vi "Engine-RPC-PWMPumpA.vi"(8 "Error In":errorcluster, 11 "DSI Reference":refnum<class "DCM-DSI.lvclass">) -> (0 "Error Out":errorcluster, 3 "DSI Reference":refnum<class "DCM-DSI.lvclass">)   [LabVIEW 2016, in "DSI-RT.lvlib"]
uses:
  DSI-RT.lvlib
  Classes/DCM-DSI/DCM-DSI.lvclass
  <vilib>/Powertrain Controls/Device Drivers/DCM/HH/FPGA/Mode.ctl
  <vilib>/Powertrain Controls/Device Drivers/DCM/HH/RT/Setup.ctl
  <vilib>/Powertrain Controls/Device Drivers/DCM/Rev0/FPGA/Digital Channel.ctl
  <vilib>/Powertrain Controls/Device Drivers/DCM/HH/RT/Angle Control.ctl
  Shared/Typedefs/Engine-RPC-PWM-Indicators.ctl
  <vilib>/addons/Software Calibration Management/xSCM/Controls/TBL1D.ctl
  <vilib>/Powertrain Controls/Device Drivers/DCM/Rev0/RT/DCM - RT.lvclass/DCM - RT.ctl
  <vilib>/Powertrain Controls/Device Drivers/DCM/HH/RT/Mode.ctl
  <vilib>/Powertrain Controls/Device Drivers/DCM/Rev0/RT/Read HH Mode.vi
  Classes/DCM-DSI/Read Channels.vi
  Classes/DCM-DSI/Read System ADC.vi
  Classes/DCM-DSI/Read dt.vi
  Classes/DCM-DSI/Write HH Command.vi
  Classes/DCM-DSI/Write HH Chans Used.vi
  Classes/DCM-DSI/Read DCM Ref.vi
  <vilib>/addons/Software Calibration Management/xSCM/CalPoint.xnode
  <vilib>/addons/Software Calibration Management/xSCM/FaultPoint.xnode
  <vilib>/Powertrain Controls/Device Drivers/DCM/Rev0/RT/DCM - RT.lvclass
  <vilib>/Powertrain Controls/Device Drivers/DCM/HH/FPGA/DCM - FPGA - HH.lvlib
  <vilib>/addons/Software Calibration Management/xSCM/ni_scm.dll
  <vilib>/addons/Software Calibration Management/xSCM/SCM-API.lvlib
  <vilib>/Powertrain Controls/Device Drivers/DCM/HH/RT/DCM - RT - HH.lvlib
  <vilib>/Powertrain Controls/Device Drivers/DCM/Rev0/FPGA/DCM - FPGA.lvlib
  Shared/DSI-Shared.lvlib
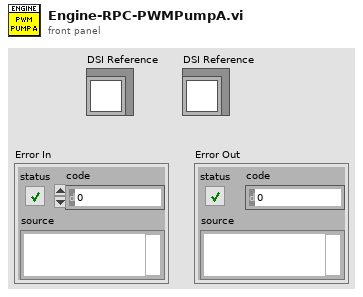
[diagram p1: front panel]
types:
  T1 = typedef "DSI-Shared.lvlib/Engine-RPC-PWM-Indicators.ctl" = cluster{"IMV":cluster{"Current_Calc":sgl, "DutyCyc_PIDOut":sgl, "DutyCyc_MaxCalc":sgl, "DutyCyc_Des":sgl}, "HPV":cluster{"Current_Calc":sgl, "DutyCyc_TblOut":sgl, "DutyCyc_MaxCalc":sgl, "DutyCyc_Des":sgl}}
  T2 = typedef "DCM - RT - HH.lvlib/Setup.ctl" = cluster{"Mode":T3, "Digital Input":T4, "Polarity":bool, "Frequency [Hz]":sgl, "Duty Cycle [%]":sgl, "TDC Offset [CAD]":sgl, "Window Start [DBTDC]":sgl, "Window End [DBTDC]":sgl, "Angles":T5[], "Skip Fire":bool, "Skip Fire Index":u8}
  T3 = typedef "DCM - FPGA - HH.lvlib/Mode.ctl" = enum8{"Off", "Direct", "Pulse Width Modulation", "Engine Position Tracking"}
  T4 = typedef "DCM - FPGA.lvlib/Digital Channel.ctl" = enum8{"Unused", "User OS", "Diff IO 1", "Diff IO 2", "Diff IO 3", "Diff IO 4", "Diff IO 5", "Diff IO 6", "Diff IO 7", "Diff IO 8", "Aux 1", "Aux 2", "Aux 3", "Aux 4", "Aux 5", "Aux 6", "Aux 7", "Aux 8", "Aux 9", "Aux 10", "Aux 11", "Aux 12", "Aux 13", "Aux 14", "Aux 15", "Aux 16"}
  T5 = typedef "DCM - RT - HH.lvlib/Angle Control.ctl" = cluster{"Enable":bool, "Location [DBTDC]":sgl, "Duration [s]":sgl}
  T6 = cluster{"PID_Kp":sgl, "PID_Ti":sgl, "PID_Td":sgl, "PID_FF":sgl, "Non-PID_FF":sgl, "PID_Min":sgl, "PID_Max":sgl}
  T7 = typedef "DCM-DSI.lvclass/Channel.ctl" = cluster{"Name":string, "Unit":string, "Value":sgl}
  T8 = typedef "DCM - RT.lvclass/System ADC.ctl" = cluster{"AI 1 [V]":sgl, "AI 2 [V]":sgl, "AI 3 [V]":sgl, "AI 4 [V]":sgl, "AI 5 [V]":sgl, "AI 6 [V]":sgl, "AI 7 [V]":sgl, "AI 8 [V]":sgl, "AI 9 [V]":sgl, "AI 10 [V]":sgl, "AI 11 [V]":sgl, "AI 12 [V]":sgl, "Temp HH 1-6 [C]":sgl, "Temp HH 7-12 [C]":sgl, "Temp DI A [C]":sgl, "Temp DI Zener A [C]":sgl, "Temp DI B [C]":sgl, "Temp DI Zener B [C]":sgl, "Temp CPU [C]":sgl, "Temp Fan Intake [C]":sgl, "Temp Secondary A [C]":sgl, "Temp Primary A [C]":sgl, "Temp Boost B [C]":sgl, "Primary Range [V]":sgl, "Primary A1A2 [V]":sgl, "Primary A3A4 [V]":sgl, "Primary B3B4 [V]":sgl, "Primary B1B2 [V]":sgl, "Secondary A1A2 [V]":sgl, "Secondary A3A4 [V]":sgl, "Secondary B3B4 [V]":sgl, "Secondary B1B2 [V]":sgl, "Ext HV A [V]":sgl, "Ext HV B [V]":sgl, "FET Driver [V]":sgl, "Fan [V]":sgl, "Battery [V]":sgl, "DRVP [V]":sgl, "Key [V]":sgl, "DI Zener A [V]":sgl, "DI Zener B [V]":sgl, "Pump Zener A [V]":sgl, "Pump Zener B [V]":sgl, "MPRD [V]":sgl}
  T9 = cluster{"IMV":cluster{"PWMFreq":sgl, "NomResistance":sgl, "DutyCyc_Max":sgl, "Min Duty Cycle":sgl, "DutyCycle_ManE":bool, "DutyCycle_Man":sgl}, "HPV":cluster{"PWMFreq":sgl, "NomResistance":sgl, "DutyCyc_Max":sgl, "Min Duty Cycle":sgl, "DutyCycle_ManE":bool, "DutyCycle_Man":sgl}}
  T10 = typedef "SCM-API.lvlib/TBL1D.ctl" = cluster{"X":sgl[], "Y":sgl[]}
  T11 = cluster{"PWMFreq":sgl, "NomResistance":sgl, "DutyCyc_Max":sgl, "Min Duty Cycle":sgl, "DutyCycle_ManE":bool, "DutyCycle_Man":sgl}
  T12 = cluster{"Current_Calc":sgl, "DutyCyc_TblOut":sgl, "DutyCyc_MaxCalc":sgl, "DutyCyc_Des":sgl}
  T13 = cluster{"Enable LS Channel":bool, "Freq [Hz]":sgl, "DutyCyc [%]":sgl}
  T14 = cluster{"Current_Calc":sgl, "DutyCyc_PIDOut":sgl, "DutyCyc_MaxCalc":sgl, "DutyCyc_Des":sgl}
  T15 = cluster{"ProportionalAction":sgl, "IntegralAction":sgl, "DerivativeAction":sgl}
  T16 = typedef "DCM - RT - HH.lvlib/Mode.ctl" = enum16{"Off", "Lowside", "Highside", "PFI", "Full H", "3-Phase"}
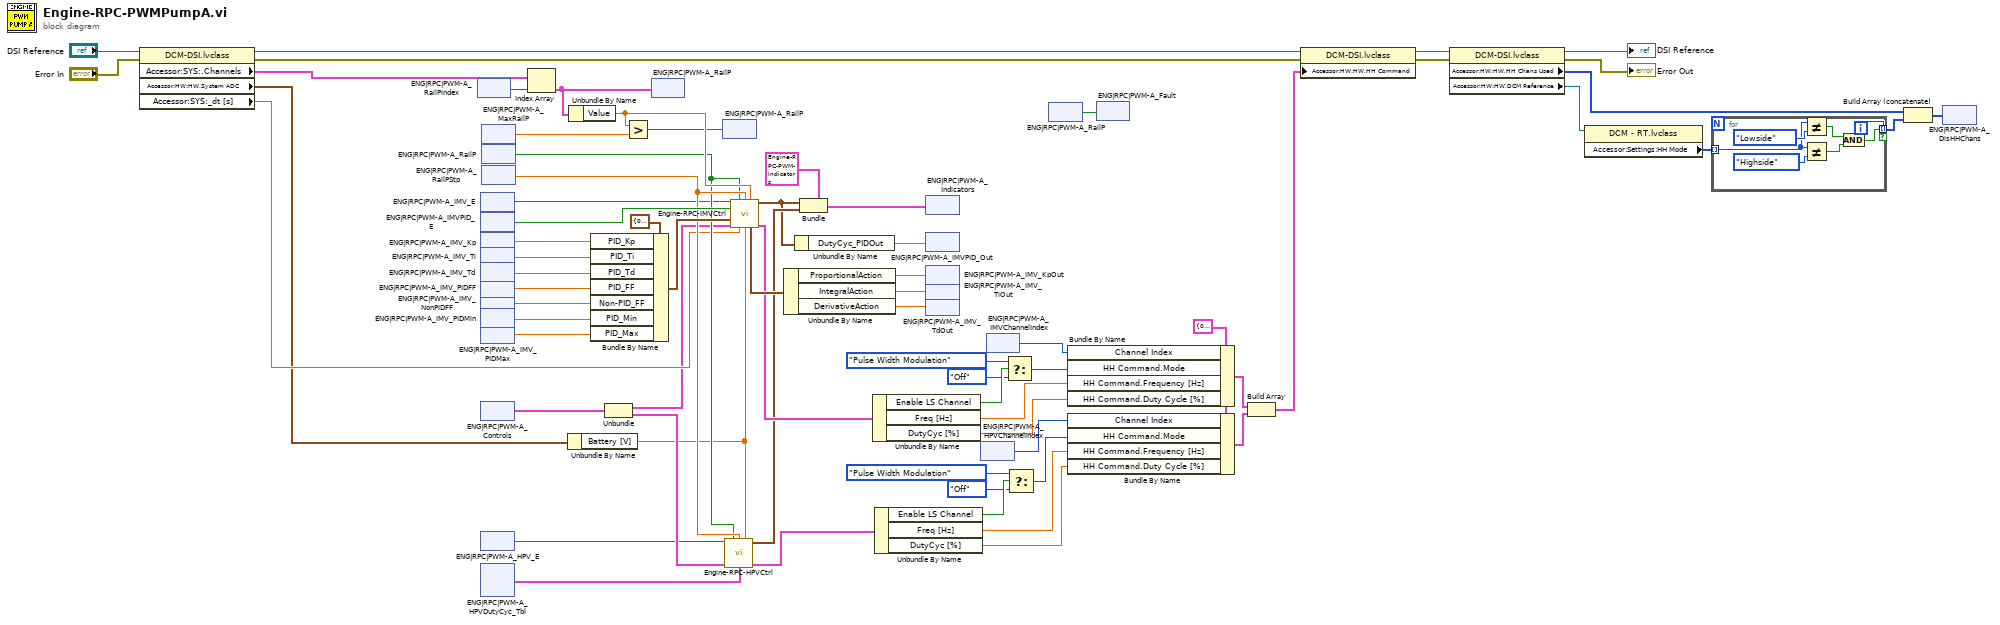
[diagram p0: block diagram]
diagram:
  w12 = cluster{"Channel Index":i32, "HH Command":T2} {"Channel Index"=0, "HH Command"={"Mode"=enum."Off", "Digital Input"=enum."Unused", "Polarity"=FALSE, "Frequency [Hz]"=0.0, "Duty Cycle [%]"=0.0, "TDC Offset [CAD]"=0.0, "Window Start [DBTDC]"=0.0, "Window End [DBTDC]"=0.0, "Angles"=[], "Skip Fire"=FALSE, "Skip Fire Index"=0}} ("HH Command")
  n1 = property class="DCM-DSI.lvclass"(reference="DSI Reference", error in="Error In") -> (reference out=w9:refnum<class "DCM-DSI.lvclass">, error out=w8:errorcluster, "Accessor:SYS:.Channels"=w13:T7[], "Accessor:HW:HW.System ADC"=w29:T8, "Accessor:SYS:_dt [s]"=w30:sgl)
  n2 = xnode "ENG|RPC|PWM-A_RailPIndex"() -> ("Value"=w39:i32)
  n3 = xnode "ENG|RPC|PWM-A_IMV_E"() -> ("Value"=w23:bool)
  n4 = xnode "ENG|RPC|PWM-A_IMVPID_E"() -> ("Value"=w36:bool)
  n5 = xnode "ENG|RPC|PWM-A_IMV_Kp"() -> ("Value"=w52:sgl)
  n6 = xnode "ENG|RPC|PWM-A_IMV_Ti"() -> ("Value"=w53:sgl)
  n7 = xnode "ENG|RPC|PWM-A_IMV_Td"() -> ("Value"=w54:sgl)
  n8 = xnode "ENG|RPC|PWM-A_IMV_PIDFF"() -> ("Value"=w55:sgl)
  n9 = xnode "ENG|RPC|PWM-A_IMV_NonPIDFF"() -> ("Value"=w56:sgl)
  n10 = xnode "ENG|RPC|PWM-A_IMV_PIDMin"() -> ("Value"=w57:sgl)
  n11 = xnode "ENG|RPC|PWM-A_IMV_PIDMax"() -> ("Value"=w58:sgl)
  n12 = xnode "ENG|RPC|PWM-A_Controls"() -> ("Value"=w22:T9)
  n13 = xnode "ENG|RPC|PWM-A_HPV_E"() -> ("Value"=w17:bool)
  n14 = xnode "ENG|RPC|PWM-A_HPVDutyCyc_Tbl"() -> ("Value"=w18:T10)
  n15 = xnode "ENG|RPC|PWM-A_MaxRailP"() -> ("Value"=w33:sgl)
  n16 = xnode "ENG|RPC|PWM-A_RailP"() -> ("Fault"=w31:bool)
  n17 = xnode "ENG|RPC|PWM-A_RailPStp"() -> ("Value"=w35:sgl)
  n18 = Index Array(array=w13, index=w39) -> (element=w38:T7)
  n19 = Unbundle By Name(w29) -> ("Battery [V]"=w19:sgl)
  n20 = Unbundle By Name(w38) -> ("Value"=w34:sgl)
  n21 = Bundle By Name(cluster=T6 {"PID_Kp"=0.0, "PID_Ti"=0.01, "PID_Td"=0.0, "PID_FF"=0.0, "Non-PID_FF"=0.0, "PID_Min"=-100.0, "PID_Max"=100.0} ("PID Settings"), "PID_Kp"=w52, "PID_Ti"=w53, "PID_Td"=w54, "PID_FF"=w55, "Non-PID_FF"=w56, "PID_Min"=w57, "PID_Max"=w58) -> (w40:T6)
  n22 = Unbundle(w22) -> ("IMV"=w21:T11, "HPV"=w20:T11)
  n23 = Greater?(x=w34, y=w33) -> (0:w32:bool)
  n24 = xnode "ENG|RPC|PWM-A_RailP"("Value"=w38) -> ()
  n25 = xnode "ENG|RPC|PWM-A_RailP"("Fault"=w32) -> ()
  n26 = call "Engine-RPC-HPVCtrl.vi"("Control Enable"=w17, "Fault Input"=w31, "RailP Setpoint"=w35, "Battery [V]"=w19, "Output Management Controls"=w20, "Open Loop DC Table"=w18) -> ("Output"=w24:T12, "LS Output"=w37:T13)  [unwired: 8 in]
  n27 = call "Engine-RPC-IMVCtrl.vi"("Control Enable"=w23, "Fault Input"=w31, "Rail Press Setpoint"=w35, "Rail Pressure"=w34, "PID Enable"=w36, "PID Settings"=w40, "Output Management Controls"=w21, "dt (s)"=w30, "Battery [V]"=w19) -> ("Output"=w14:T14, "PID_Action_Output"=w59:T15, "LS Output"=w45:T13)  [unwired: 4 in]
  n28 = Unbundle By Name(w59) -> ("ProportionalAction"=w2:sgl, "IntegralAction"=w3:sgl, "DerivativeAction"=w4:sgl)
  n29 = Unbundle By Name(w14) -> ("DutyCyc_PIDOut"=w1:sgl)
  n30 = Bundle(cluster=T1 {"IMV"={"Current_Calc"=0.0, "DutyCyc_PIDOut"=0.7671859, "DutyCyc_MaxCalc"=0.0, "DutyCyc_Des"=0.7671859}, "HPV"={"Current_Calc"=0.0, "DutyCyc_TblOut"=0.7671859, "DutyCyc_MaxCalc"=0.0, "DutyCyc_Des"=0.7671859}} ("PWM-B_Indicators"), "IMV"=w14, "HPV"=w24) -> (w5:T1)
  n31 = Unbundle By Name(w45) -> ("Enable LS Channel"=w50:bool, "Freq [Hz]"=w48:sgl, "DutyCyc [%]"=w47:sgl)
  n32 = Unbundle By Name(w37) -> ("Enable LS Channel"=w46:bool, "Freq [Hz]"=w27:sgl, "DutyCyc [%]"=w26:sgl)
  n33 = xnode "ENG|RPC|PWM-A_Indicators"("Value"=w5) -> ()
  n34 = xnode "ENG|RPC|PWM-A_IMVPID_Out"("Value"=w1) -> ()
  n35 = xnode "ENG|RPC|PWM-A_IMV_KpOut"("Value"=w2) -> ()
  n36 = xnode "ENG|RPC|PWM-A_IMV_TiOut"("Value"=w3) -> ()
  n37 = xnode "ENG|RPC|PWM-A_IMV_TdOut"("Value"=w4) -> ()
  n38 = xnode "ENG|RPC|PWM-A_HPVChannelIndex"() -> ("Value"=w15:i32)
  n39 = xnode "ENG|RPC|PWM-A_IMVChannelIndex"() -> ("Value"=w16:i32)
  n40 = Select(t=Mode."Pulse Width Modulation" ("Mode"), s=w50, f=Mode."Off" ("Mode")) -> (s? t:f=w49:T3)
  n41 = Select(t=Mode."Pulse Width Modulation" ("Mode"), s=w46, f=Mode."Off" ("Mode")) -> (s? t:f=w28:T3)
  n42 = xnode "ENG|RPC|PWM-A_RailP"() -> ("Fault"=w10:bool)
  n43 = Bundle By Name(cluster=w12, "Channel Index"=w16, "HH Command.Mode"=w49, "HH Command.Frequency [Hz]"=w48, "HH Command.Duty Cycle [%]"=w47) -> (w11:cluster{"Channel Index":i32, "HH Command":T2})
  n44 = Bundle By Name(cluster=w12, "Channel Index"=w15, "HH Command.Mode"=w28, "HH Command.Frequency [Hz]"=w27, "HH Command.Duty Cycle [%]"=w26) -> (w25:cluster{"Channel Index":i32, "HH Command":T2})
  n45 = xnode "ENG|RPC|PWM-A_Fault"("Value"=w10) -> ()
  n46 = Build Array(w11, w25) -> (w7:cluster{"Channel Index":i32, "HH Command":T2}[])
  n47 = property class="DCM-DSI.lvclass"(reference=w9, error in=w8, "Accessor:HW:HW.HH Command"=w7) -> (reference out=w66:refnum<class "DCM-DSI.lvclass">, error out=w65:errorcluster)
  n48 = property class="DCM-DSI.lvclass"(reference=w66, error in=w65) -> (reference out=→"DSI Reference":refnum<class "DCM-DSI.lvclass">, error out=→"Error Out":errorcluster, "Accessor:HW:HW.HH Chans Used"=w61:i32[], "Accessor:HW:HW.DCM Reference"=w62:refnum<class "DCM - RT.lvclass">)
  n49 = property class="DCM - RT.lvclass"(reference=w62) -> ("Accessor:Settings:HH Mode"=w64:T16[])  [unwired: 1 in, 2 out]
  n50 = for {
    tunnel: [w76] -> w60 mode=indexing if=w74
    tunnel: w64 -> [w71] mode=indexing
    i -> [w76]
    n51 = Not Equal?(x=w71, y=Mode."Lowside" ("Mode")) -> (x != y?=w73:bool)
    n52 = Not Equal?(x=w71, y=Mode."Highside" ("Mode")) -> (x != y?=w72:bool)
    n53 = And(x=w73, y=w72) -> (x .and. y?=w74:bool)
  }
  n54 = Build Array (concatenate)(w61, w60) -> (w63:i32[])
  n55 = xnode "ENG|RPC|PWM-A_DisHHChans"("Value"=w63) -> ()
